vi "Airheater Model subsystem.vi"(0 "u [V]":dbl format="%#_13g", 1 "K [C/V]":dbl=3.5, 2 "T_enviroment [C]":dbl=21.0, 3 "T_initial [C]":dbl=21.0, 4 "Time constant [s]":dbl=22.0, 5 "Delay [s]":dbl=3.0) -> (16 "T_out [C]":dbl)   [LabVIEW 2019]
uses:
  <vilib>/Simulation/Implementation/Shared/SIMSCR Execution Mode.ctl
  <vilib>/Simulation/Scripting/Companion Diagram/SimConfigNode/SimParams.ctl
  <vilib>/Simulation/Scripting/Companion Diagram/SimConfigNode/_simSolvers.ctl
  <vilib>/Simulation/Param Hierarchy/Typedefs/SIMPH Param Control Actions.ctl
  <vilib>/Simulation/Implementation/Shared/SIM limit type.ctl
  <vilib>/Simulation/Implementation/Shared/NILVSim_ParamChanged.vi
  <vilib>/Simulation/Implementation/Shared/NILVSIM_BeginStep.vi
  <vilib>/Simulation/ContinuousLinear/Implementation/NILVSim Integrator new.llb/SIM Integrator distributor (scalar).vi
  <vilib>/Simulation/ContinuousLinear/Implementation/NILVSim Transport Delay.llb/SIM Transport Delay Distributor (scalar).vi
  <vilib>/Simulation/ContinuousLinear/Implementation/NILVSim Transport Delay.llb/SIM Transport Delay Collector (scalar).vi
  <vilib>/Simulation/ContinuousLinear/Implementation/NILVSim Integrator new.llb/SIM Integrator collector (scalar).vi
  <vilib>/Simulation/Implementation/Shared/NILVSim_Manager.vi
  <vilib>/Utility/error.llb/Clear Errors.vi
  <vilib>/Simulation/Implementation/Shared/NILVSim_FinalizeModel.vi
  <vilib>/Simulation/Implementation/Shared/SIM Unbundle Sim Info.vi
  <vilib>/Simulation/Implementation/Shared/SIMSH Read Queue.vi
  <vilib>/Simulation/Implementation/Shared/NILVSim_Initialize.vi
  <vilib>/Simulation/Utility/Implementation/NILVSim Get Time and IsAcceptedStep.vi
  <vilib>/Simulation/Implementation/Shared/NILVSim_GetModelError.vi
  <vilib>/Simulation/Implementation/Shared/SIM SimErrorHandler.vi
  <vilib>/Simulation/Implementation/Shared/SIM Bundle Sim Info.vi
  <vilib>/Simulation/Scripting/Companion Diagram/SimConfigNode/SimDog.xnode
  <vilib>/Simulation/Implementation/XNodeFramework/SimXNode/SimX.xnode
  <vilib>/Simulation/ContinuousLinear/Implementation/NILVSim Integrator new.llb/SIM Integrator (scalar).vi
  <vilib>/Simulation/ContinuousLinear/Implementation/NILVSim Transport Delay.llb/SIM Transport Delay Indirect (scalar).vi
  <vilib>/Simulation/Implementation/Shared/NI_SIM_Implementation.lvlib
panel:
  # "Simulation Output"
  # "Simulation Variables"
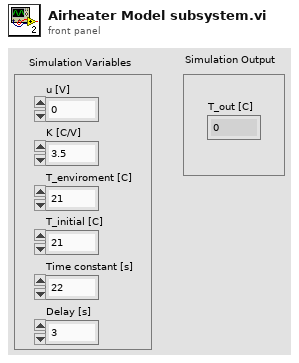
[diagram p1: front panel]
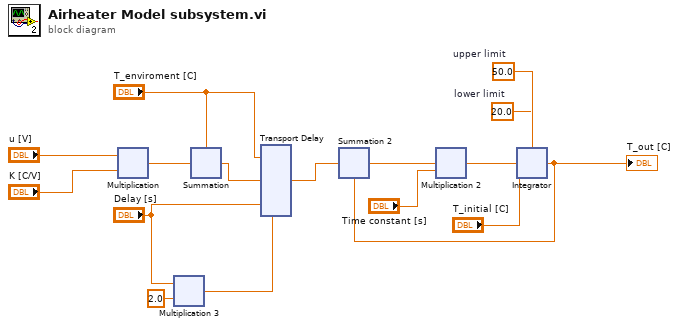
[diagram p0: block diagram]
diagram:
  w9 = 20.0  # lower limit
  w10 = 50.0  # upper limit
  n1 = xnode ("Multiplication")("Operand1"="u [V]", "Operand2"="K [C/V]") -> ("Result"=w14:dbl)
  n2 = xnode ("Multiplication 3")("Operand1"="Delay [s]", "Operand2"=2.0) -> ("Result"=w1:dbl)
  n3 = xnode ("Summation")("Operand1"="T_enviroment [C]", "Operand2"=w14) -> ("Result"=w3:dbl)
  n4 = xnode "Transport Delay"("initial condition"="T_enviroment [C]", "max delay (s)"=w1, "input"=w3, "delay (s)"="Delay [s]") -> ("output"=w13:dbl)  [unwired: 1 in]
  n5 = xnode ("Summation 2")("Operand1"=w13, "Operand2"=w6) -> ("Result"=w12:dbl)
  n6 = xnode ("Multiplication 2")("Operand1"=w12, "Operand2"="Time constant [s]") -> ("Result"=w8:dbl)
  n7 = xnode ("Integrator")("upper limit"=w10, "input"=w8, "initial condition"="T_initial [C]", "lower limit"=w9) -> ("output"=w6:dbl)  [unwired: 6 in, 2 out]
  "T_out [C]" <- w6
